vi "Async Loop Control.vi"(7 "Action":T18, 8 "error in (no error)":errorcluster, 10 "RT Data In":T1 {"Label Transfer Config"."Block Data Refs"."Data Reference" format="%.0x"; "Status Config"."HWOut Dur Ref" format="%.0x"; "Status Config"."HWIn Dur Ref" format="%.0x"; "Status Config"."Error Data Ref" format="%.0x"; "HWOutput Channels"."Labels Settings"."Label" format="%.0o"; "HWInput Channels"."Labels Settings"."Label" format="%.0o"}) -> (0 "error out":errorcluster, 2 "RT Data Out":T1 {"Label Transfer Config"."Block Data Refs"."Data Reference" format="%.0x"; "Status Config"."HWOut Dur Ref" format="%.0x"; "Status Config"."HWIn Dur Ref" format="%.0x"; "Status Config"."Error Data Ref" format="%.0x"; "HWOutput Channels"."Labels Settings"."Label" format="%.0o"; "HWInput Channels"."Labels Settings"."Label" format="%.0o"})   [LabVIEW 2015, in "AIT 429 Engine.lvlib"]
doc: "Controls the Async Loops (Meas Write/Read, Char Write/Read) according to the action input."
uses:
  AIT 429 Engine.lvlib
  RT Controls/RT Data.ctl
  RT Controls/RT HW Channel.ctl
  RT Controls/RT Label Settings.ctl
  Shared/Controls and Global/Label.ctl
  Shared/Controls and Global/transferPeriod.ctl
  RT Controls/Driver Data.ctl
  RT Controls/RT Word Settings.ctl
  <vilib>/NI Veristand/Custom Device API/Block Data Reference.ctl
  <vilib>/NI Veristand/Custom Device API/Data Reference.ctl
  RT Controls/RT Param Setting.ctl
  Shared/Controls and Global/Start Bit.ctl
  Shared/Controls and Global/Number of Bits.ctl
  Shared/Controls and Global/TransferType.ctl
  RT Controls/Error Qs.ctl
  RT Controls/Status Channels Config.ctl
  RT Controls/FIFO.ctl
  RT Controls/Label Transfer Config.ctl
  RT Controls/Async Loop Control Enum.ctl
  Shared/AIT 429 Shared.lvlib
  <vilib>/NI Veristand/Custom Device API/Custom Device API.lvlib
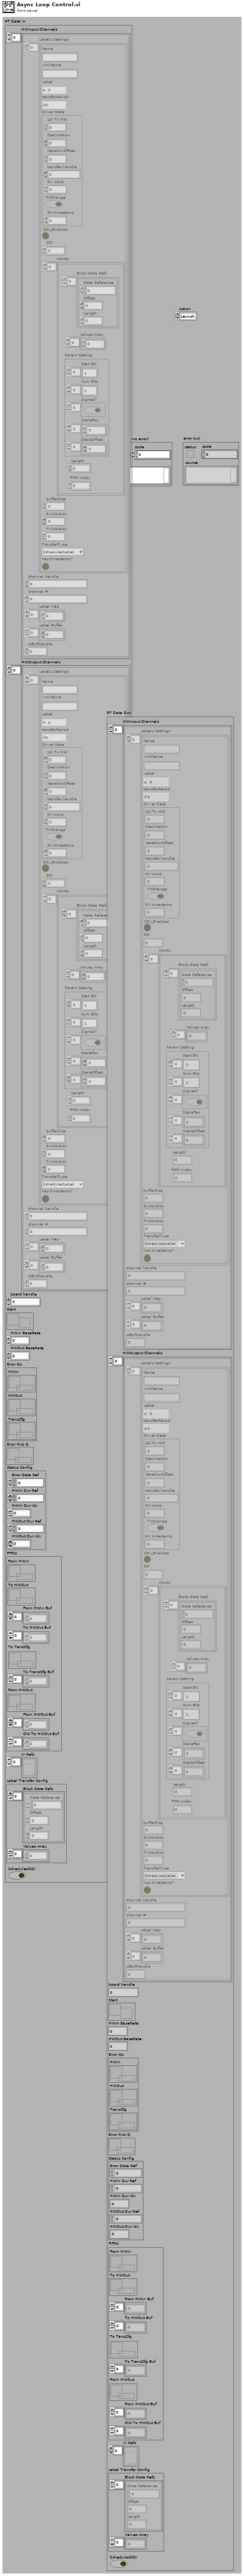
[diagram p1: front panel]
types:
  T1 = typedef "AIT 429 Engine.lvlib/RT Data.ctl" = cluster{"HWInput Channels":T2[], "HWOutput Channels":T2[], "board handle":u32, "Start":refnum<notifier>, "HWIn BaseRate":i64, "HWOut BaseRate":i64, "Error Qs":T14, "Error Pub Q":refnum<queue>, "Status Config":T15, "FIFOs":T16, "VI Refs":refnum<vi>[], "Label Transfer Config":T17, "ScheduledSDI":bool}
  T2 = typedef "AIT 429 Engine.lvlib/RT HW Channel.ctl" = cluster{"Labels Settings":T3[], "channel handle":u32, "channel #":u16, "Label Map":i32[], "Label Buffer":u32[], "rdBufHandle":u32}
  T3 = typedef "AIT 429 Engine.lvlib/RT Label Settings.ctl" = cluster{"Name":string, "xmlName":string, "Label":T4, "transferPeriod":T5, "Driver Data":T6, "SDI_Enabled":bool, "SDI":u8, "Words":T7[], "bufferSize":u32, "RxWordIdx":i32, "TxWordIdx":i32, "TransferType":T13, "has timestamp?":bool}
  T4 = typedef "AIT 429 Shared.lvlib/Label.ctl" = u8
  T5 = typedef "AIT 429 Shared.lvlib/transferPeriod.ctl" = u32
  T6 = typedef "AIT 429 Engine.lvlib/Driver Data.ctl" = cluster{"Lbl Tx Hdl":u32, "Decimation":i32, "IterationOffset":i32, "transfer handle":u32, "RX Word":u32, "TXChange":bool, "RX timestamp":dbl}
  T7 = typedef "AIT 429 Engine.lvlib/RT Word Settings.ctl" = cluster{"Block Data Refs":T8[], "Values Array":dbl[], "Length":i32, "FIFO Index":i32, "Param Setting":T10}
  T8 = typedef "Custom Device API.lvlib/Block Data Reference.ctl" = cluster{"Data Reference":T9, "Offset":u64, "Length":u64}
  T9 = typedef "Custom Device API.lvlib/Data Reference.ctl" = i32
  T10 = typedef "AIT 429 Engine.lvlib/RT Param Setting.ctl" = cluster{"Start Bit":T11[], "Num Bits":T12[], "Signed?":bool[], "ScaleFac":dbl[], "ScaleOffset":dbl[]}
  T11 = typedef "AIT 429 Shared.lvlib/Start Bit.ctl" = i32
  T12 = typedef "AIT 429 Shared.lvlib/Number of Bits.ctl" = i32
  T13 = typedef "AIT 429 Shared.lvlib/TransferType.ctl" = enum16{"ScheduledLabel", "Acyclic", "Block", "Strobe"}
  T14 = typedef "AIT 429 Engine.lvlib/Error Qs.ctl" = cluster{"HWIn":refnum<queue>, "HWOut":refnum<queue>, "TransCfg":refnum<queue>}
  T15 = typedef "AIT 429 Engine.lvlib/Status Channels Config.ctl" = cluster{"Error Data Ref":T9, "HWIn Dur Ref":T9, "HWIn Dur Idx":i32, "HWOut Dur Ref":T9, "HWOut Dur Idx":i32}
  T16 = typedef "AIT 429 Engine.lvlib/FIFO.ctl" = cluster{"From HWIn":refnum<k33>, "To HWOut":refnum<k33>, "From HWIn Buf":dbl[], "To HWOut Buf":dbl[], "To TansCfg":refnum<k33>, "To TransCfg Buf":dbl[], "From HWOut":refnum<k33>, "From HWOut Buf":dbl[], "Old To HWOut Buf":dbl[]}
  T17 = typedef "AIT 429 Engine.lvlib/Label Transfer Config.ctl" = cluster{"Block Data Refs":T8[], "Values Array":dbl[]}
  T18 = typedef "AIT 429 Engine.lvlib/Async Loop Control Enum.ctl" = enum16{"Launch", "Start", "Stop"}
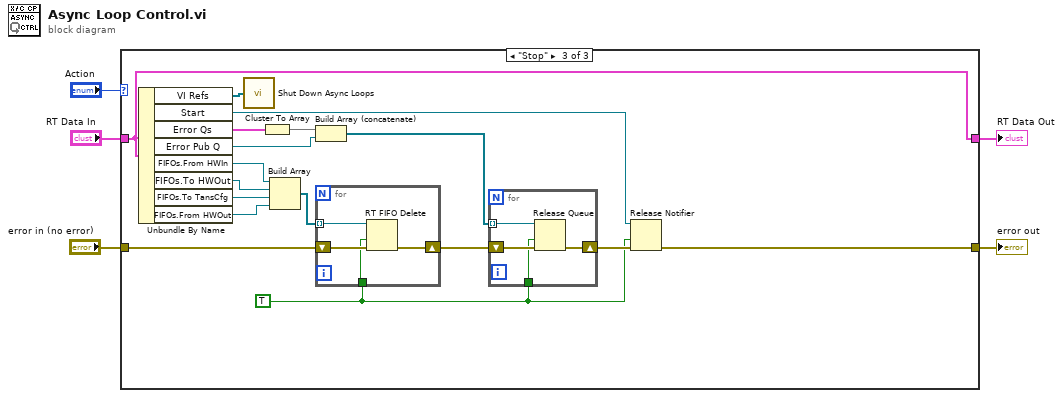
[diagram p0: block diagram]
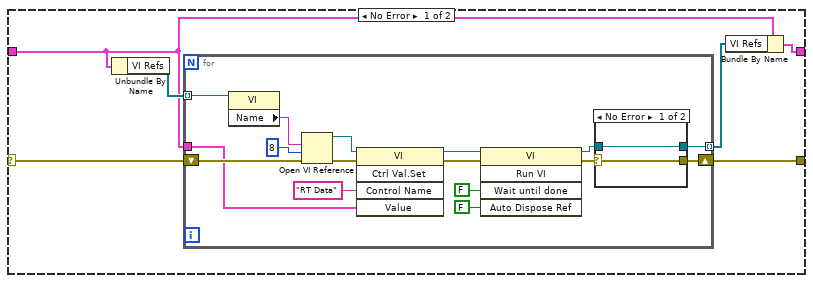
[diagram p3: hidden frame]
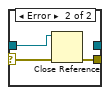
[diagram p4: hidden frame]
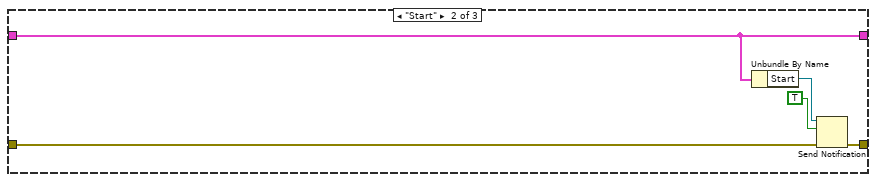
[diagram p5: hidden frame]
diagram:
  n1 = case shown="\"Stop\"" "Action" {
    tunnel: [w9 w40 w47] -> w5
    tunnel: "error in (no error)" -> [w8 w42 w49]
    tunnel: "RT Data In" -> [w7 w39 w51]
    tunnel: [w6 w39 w51] -> w1
    frame "Launch", Default {
      n2 = case shown="Error" w8 {
        selector: w8 -> [w15 w38]
        tunnel: [w14 w38] -> w9
        tunnel: w7 -> [w12 w37]
        tunnel: [w10 w37] -> w6
        frame No Error {
          n3 = Unbundle By Name(w12) -> ("VI Refs"=w13:refnum<vi>[])
          n4 = for {
            shift-right: [w28] -> w14
            shift-left: w15 -> [w31]
            tunnel: w13 -> [w30] mode=indexing
            tunnel: w12 -> [w16]
            tunnel: [w29] -> w11 mode=indexing
            n5 = property class="VI"(reference=w30) -> ("Name"=w27:string)  [unwired: 1 in, 2 out]
            n6 = Open VI Reference(vi path=w27, options=8, error in (no error)=w31) -> (vi reference=w19:refnum<vi>, error out=w20:errorcluster)  [unwired: 3 out]
            n7 = invoke class="VI" method="Ctrl Val.Set"(reference=w19, error in=w20, "Control Name"="RT Data", "Value"=w16) -> (reference out=w21:refnum<vi>, error out=w17:errorcluster)  [unwired: 1 in, 3 out]
            n8 = invoke class="VI" method="Run VI"(reference=w21, error in=w17, "Wait until done"=FALSE ("Wait Until Done"), "Auto Dispose Ref"=FALSE ("Auto Dispose Reference")) -> (reference out=w22:refnum<vi>, error out=w23:errorcluster)  [unwired: 1 in, 3 out]
            n9 = case shown="No Error" w23 {
              selector: w23 -> [w33 w36]
              tunnel: w22 -> [w32 w35]
              tunnel: [w33 w34] -> w28
              tunnel: [w32 _] -> w29
              frame No Error {
              }
              frame Error {
                n10 = Close Reference(reference=w35, error in (no error)=w36) -> (error out=w34:errorcluster)
              }
            }
          }
          n11 = Bundle By Name(cluster=w12, "VI Refs"=w11) -> (w10:T1)
        }
        frame Error {
        }
      }
    }
    frame "Start" {
      n12 = Unbundle By Name(w39) -> ("Start"=w43:refnum<notifier>)
      n13 = Send Notification(notification=TRUE, notifier=w43, error in (no error)=w42) -> (error out=w40:errorcluster)  [unwired: 1 out]
    }
    frame "Stop" {
      w46 = TRUE ("force destroy? (F)")
      n14 = Unbundle By Name(w51) -> ("VI Refs"=w50:refnum<vi>[], "Start"=w55:refnum<notifier>, "Error Qs"=w60:T14, "Error Pub Q"=w57:refnum<queue>, "FIFOs.From HWIn"=w54:refnum<k33>, "FIFOs.To HWOut"=w53:refnum<k33>, "FIFOs.To TansCfg"=w45:refnum<k33>, "FIFOs.From HWOut"=w44:refnum<k33>)
      n15 = call "Shut Down Async Loops.vi"("VI Refs"=w50) -> ()
      n16 = Cluster To Array(cluster=w60) -> (array=w59:refnum<queue>[])
      n17 = Build Array(w54, w53, w45, w44) -> (w52:refnum<k33>[])
      n18 = Build Array (concatenate)(w59, w57) -> (w58:refnum<queue>[])
      n19 = for {
        shift-right: [w63] -> w48
        shift-left: w49 -> [w64]
        tunnel: w52 -> [w62] mode=indexing
        tunnel: w46 -> [w61]
        n20 = RT FIFO Delete(0:w62, 2:w61, 3:w64) -> (11:w63:errorcluster)
      }
      n21 = for {
        shift-right: [w67] -> w56
        shift-left: w48 -> [w68]
        tunnel: w58 -> [w66] mode=indexing
        tunnel: w46 -> [w65]
        n22 = Release Queue(queue=w66, force destroy? (F)=w65, error in (no error)=w68) -> (error out=w67:errorcluster)  [unwired: 2 out]
      }
      n23 = Release Notifier(notifier=w55, force destroy? (F)=w46, error in (no error)=w56) -> (error out=w47:errorcluster)  [unwired: 2 out]
    }
  }
  "error out" <- w5
  "RT Data Out" <- w1
